vi "niRFUtil FTW Compute RBW Min Sampling Rate.vi"(0 "Type":T2=enum."Gaussian", 5 "Center Frequency (Hz)":dbl format="%^.2e", 7 "Bandwidth (Hz)":T3 format="%^.3e", 9 "Minimum Selectivity (dB)":dbl=70.0 format="%.2f", 11 "Alpha":T1=0.22 format="%.3g") -> (4 "Min Sampling Rate (Hz)":dbl format="%^.2e", 6 "Filter Bandwidth (Hz)":dbl format="%^.2e")   [LabVIEW 2015, in "niRFUtil.lvlib"]
doc: "(c) Copyright 2006, National Instruments, Inc. This VI may not be duplicated, sold, or distributed without written consent from National Instruments."
uses:
  niRFUtil.lvlib
  Includes/niRFUtil INC RBW Filter Bandwidth.ctl
  Includes/niRFUtil INC RBW Filter Type (Time Domain).ctl
  Includes/niRFUtil INC RRC Filter Alpha.ctl
  Includes/niRFUtil INC RBW Filter Type (Freq Domain).ctl
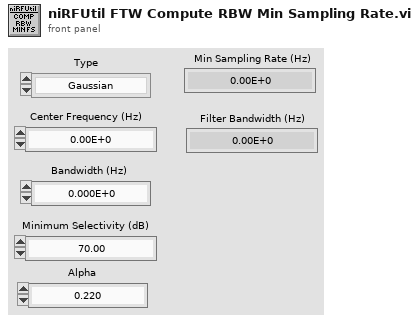
[diagram p1: front panel]
types:
  T1 = typedef "niRFUtil.lvlib/niRFUtil INC RRC Filter Alpha.ctl" = dbl
  T2 = typedef "niRFUtil.lvlib/niRFUtil INC RBW Filter Type (Time Domain).ctl" = enum16{"None", "Gaussian", "Flat", "Synch Tuned - 4", "Synch Tuned - 5", "RRC"}
  T3 = typedef "niRFUtil.lvlib/niRFUtil INC RBW Filter Bandwidth.ctl" = dbl
  T4 = typedef "niRFUtil.lvlib/niRFUtil INC RBW Filter Type (Freq Domain).ctl" = enum16{"FFT Based", "Gaussian", "Flat", "Synch Tuned - 4", "Synch Tuned - 5"}
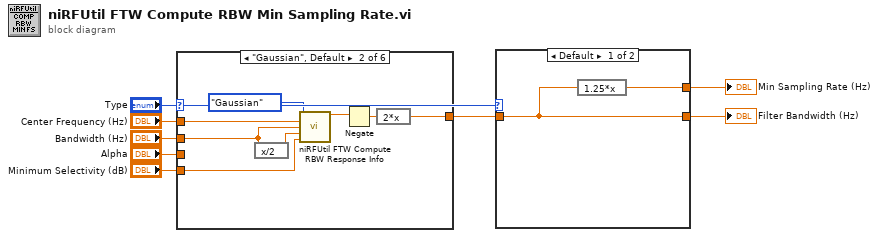
[diagram p0: block diagram]
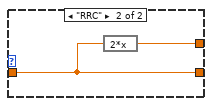
[diagram p2: hidden frame]
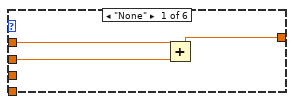
[diagram p3: hidden frame]
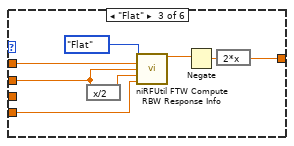
[diagram p4: hidden frame]
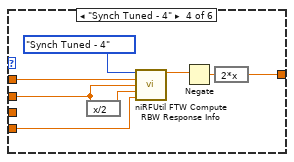
[diagram p5: hidden frame]
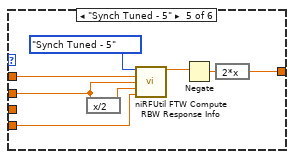
[diagram p6: hidden frame]
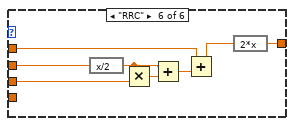
[diagram p7: hidden frame]
diagram:
  n1 = case shown="\"Gaussian\", Default" "Type" {
    tunnel: "Center Frequency (Hz)" -> [w11 w19 w27 w35 w43 w46]
    tunnel: "Bandwidth (Hz)" -> [w9 w17 w26 w34 w42 w51]
    tunnel: "Minimum Selectivity (dB)" -> [_ w18 w24 w32 w40 _]
    tunnel: [w10 w14 w22 w30 w38 w44] -> w2
    tunnel: "Alpha" -> [_ _ _ _ _ w50]
    frame "None" {
      n2 = Add(x=w11, y=w9) -> (x+y=w10:T3)
    }
    frame "Gaussian", Default {
      n3 = expression code="x/2"(w17) -> (w16:T3)
      n4 = call "niRFUtil FTW Compute RBW Response Info.vi"("Type"=niRFUtil_INC_RBW_Filter_Type_(Freq_Domain)."Gaussian", "Center Frequency (Hz)"=w19, "Bandwidth (Hz)"=w17, "df (Hz)"=w16, "Minimum Selectivity (dB)"=w18) -> ("Start Frequency (Hz)"=w12:sgl)  [unwired: 10 in]
      n5 = Negate(x=w12) -> (-x=w15:sgl)
      n6 = expression code="2*x"(w15) -> (w14:sgl)
    }
    frame "Flat" {
      n7 = expression code="x/2"(w26) -> (w25:T3)
      n8 = call "niRFUtil FTW Compute RBW Response Info.vi"("Type"=niRFUtil_INC_RBW_Filter_Type_(Freq_Domain)."Flat", "Center Frequency (Hz)"=w27, "Bandwidth (Hz)"=w26, "df (Hz)"=w25, "Minimum Selectivity (dB)"=w24) -> ("Start Frequency (Hz)"=w21:sgl)  [unwired: 10 in]
      n9 = Negate(x=w21) -> (-x=w23:sgl)
      n10 = expression code="2*x"(w23) -> (w22:sgl)
    }
    frame "Synch Tuned - 4" {
      n11 = expression code="x/2"(w34) -> (w33:T3)
      n12 = call "niRFUtil FTW Compute RBW Response Info.vi"("Type"=niRFUtil_INC_RBW_Filter_Type_(Freq_Domain)."Synch Tuned - 4", "Center Frequency (Hz)"=w35, "Bandwidth (Hz)"=w34, "df (Hz)"=w33, "Minimum Selectivity (dB)"=w32) -> ("Start Frequency (Hz)"=w29:sgl)  [unwired: 10 in]
      n13 = Negate(x=w29) -> (-x=w31:sgl)
      n14 = expression code="2*x"(w31) -> (w30:sgl)
    }
    frame "Synch Tuned - 5" {
      n15 = expression code="x/2"(w42) -> (w41:T3)
      n16 = call "niRFUtil FTW Compute RBW Response Info.vi"("Type"=niRFUtil_INC_RBW_Filter_Type_(Freq_Domain)."Synch Tuned - 5", "Center Frequency (Hz)"=w43, "Bandwidth (Hz)"=w42, "df (Hz)"=w41, "Minimum Selectivity (dB)"=w40) -> ("Start Frequency (Hz)"=w36:sgl)  [unwired: 10 in]
      n17 = Negate(x=w36) -> (-x=w39:sgl)
      n18 = expression code="2*x"(w39) -> (w38:sgl)
    }
    frame "RRC" {
      n19 = expression code="x/2"(w51) -> (w48:T3)
      n20 = Multiply(x=w48, y=w50) -> (x*y=w49:T3)
      n21 = Add(x=w48, y=w49) -> (x+y=w47:T3)
      n22 = Add(x=w46, y=w47) -> (x+y=w45:T3)
      n23 = expression code="2*x"(w45) -> (w44:T3)
    }
  }
  n24 = case shown="Default" "Type" {
    tunnel: [w53 w55] -> w3
    tunnel: w2 -> [w53 w55]
    tunnel: [w52 w54] -> w1
    frame Default {
      n25 = expression code="1.25*x"(w53) -> (w52:T3)
    }
    frame "RRC" {
      n26 = expression code="2*x"(w55) -> (w54:T3)
    }
  }
  "Min Sampling Rate (Hz)" <- w1
  "Filter Bandwidth (Hz)" <- w3
